vi "Unibot - State Machine Controller.vi"(5 "Up Optimal Gain":dbl[](array[numeric])=[-16.4615, -16.2422, -3.1287, -2.0658], 7 "Setpoint Theta":dbl(knob) scale=-0.1..0.1, 8 "Enable":bool, 9 "Kill":bool, 10 "Setpoint V":dbl(knob) scale=-0.1..0.1, 11 "States":dbl[](array[numeric])=[-0.0012566370614359172, -0.8117875416876026, 0.0, 0.0]) -> (0 "Status":string="Kill", 2 "Control Effort":dbl=-0.1425196371146851)   [LabVIEW 2012]
uses:
  Code/LabVIEW/Real-Time/Demos/cRIO Motor Control/Unibot/Unibot - States.ctl
  <vilib>/addons/Control Design/_Implementation/CD State Feedback Controller (Single Output).vi
  <vilib>/addons/Control Design/_Implementation/NI_CD_Implementation.lvlib
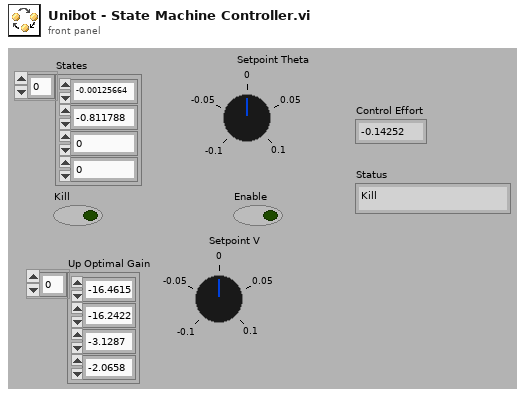
[diagram p1: front panel]
types:
  T1 = typedef "Unibot - States.ctl" = enum16{"Idle", "Balance", "Emergency"}
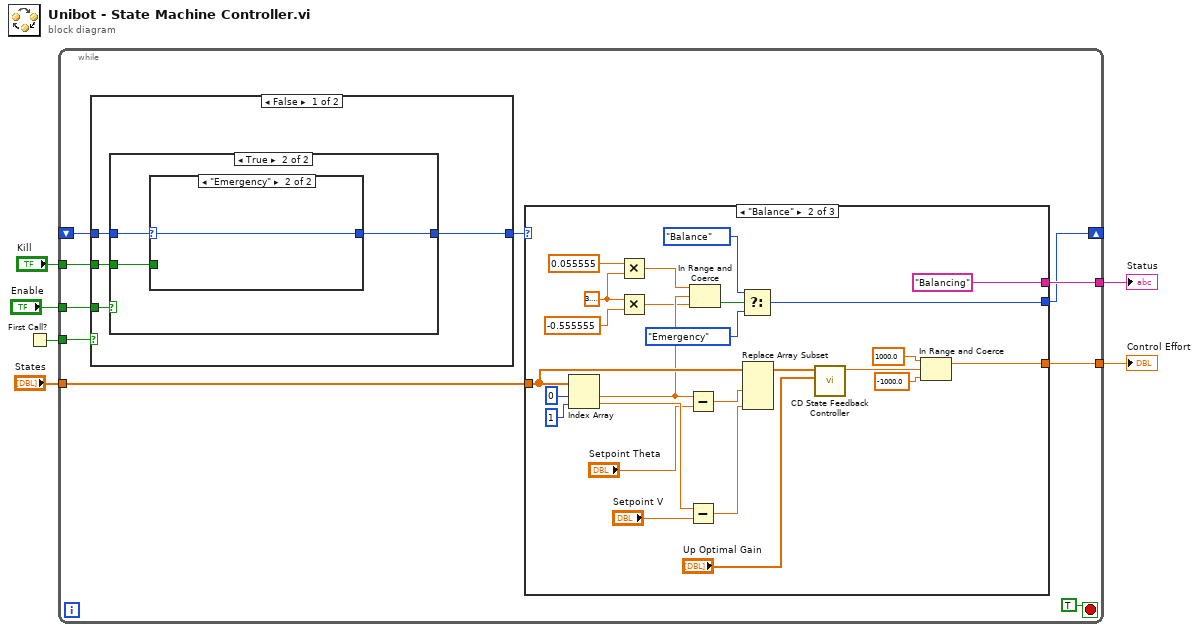
[diagram p0: block diagram]
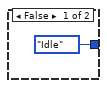
[diagram p2: hidden frame]
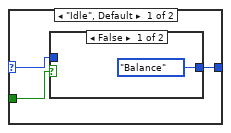
[diagram p3: hidden frame]
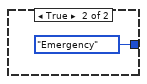
[diagram p4: hidden frame]
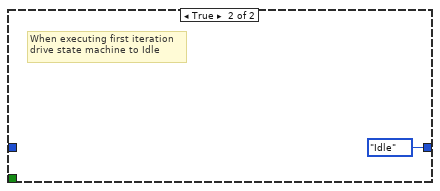
[diagram p5: hidden frame]
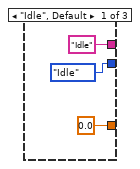
[diagram p6: hidden frame]
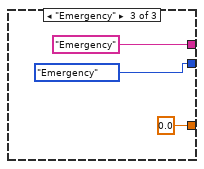
[diagram p7: hidden frame]
diagram:
  n1 = First Call?() -> (First Call?: T/F=w2:bool)
  n2 = while {
    tunnel: "States" -> [w15]
    tunnel: [w11] -> w5
    shift-right: [w10] -> _
    shift-left: _ -> [w12]
    tunnel: [w14] -> w4
    tunnel: "Kill" -> [w13]
    tunnel: w2 -> [w8]
    tunnel: "Enable" -> [w7]
    stop <- TRUE stop-if-true
    n3 = case shown="False" w8 {
      tunnel: w13 -> [w20 _]
      tunnel: w12 -> [w19 _]
      tunnel: [w18 Unibot_-_States."Idle" ("Enum")] -> w9
      tunnel: w7 -> [w17 _]
      frame False {
        n4 = case shown="True" w17 {
          tunnel: w20 -> [_ w24]
          tunnel: [Unibot_-_States."Idle" ("Enum") w23] -> w18
          tunnel: w19 -> [_ w22]
          frame False {
          }
          frame True {
            n5 = case shown="\"Emergency\"" w22 {
              selector: w22 -> [w26 w30]
              tunnel: w24 -> [w27 _]
              tunnel: [w25 w30] -> w23
              frame "Idle", Default {
                n6 = case shown="False" w27 {
                  tunnel: [Unibot_-_States."Balance" ("Enum") Unibot_-_States."Emergency" ("Enum")] -> w25
                  tunnel: w26 -> [_ _]
                  frame False {
                  }
                  frame True {
                  }
                }
              }
              frame "Emergency" {
              }
            }
          }
        }
      }
      frame True {
        # "When executing first iteration\ndrive state machine to Idle"
      }
    }
    n7 = case shown="\"Balance\"" w9 {
      tunnel: w15 -> [_ w52 _]
      tunnel: [0.0 w46 0.0] -> w11
      tunnel: [Unibot_-_States."Idle" ("Enum") w59 Unibot_-_States."Emergency" ("Enum")] -> w10
      tunnel: ["Idle" "Balancing" "Emergency"] -> w14
      frame "Idle", Default {
      }
      frame "Balance" {
        w44 = 3.141592653589793 ("Setpoint")
        n8 = Index Array(array=w52, index #1=0 ("index"), index #2=1 ("index")) -> (element #1=w51:dbl, element #2=w54:dbl)
        n9 = Multiply(x=0.055555, y=w44) -> (x*y=w42:dbl)
        n10 = Multiply(x=w44, y=-0.555555) -> (x*y=w40:dbl)
        n11 = Subtract(x=w51, y="Setpoint Theta") -> (x-y=w55:dbl)
        n12 = Subtract(x=w54, y="Setpoint V") -> (x-y=w53:dbl)
        n13 = In Range and Coerce(upper limit=w42, x=w51, lower limit=w40) -> (In Range?=w39:bool)  [unwired: 1 out]
        n14 = Select(t=Unibot_-_States."Balance" ("Enum"), s=w39, f=Unibot_-_States."Emergency" ("Enum")) -> (s? t:f=w59:T1)
        n15 = Replace Array Subset(array=w52, new element #1=w55, new element #2=w53) -> (w58:dbl[])  [unwired: 2 in]
        n16 = call-poly <vilib>:"CD State Feedback Controller.vi"("Controller Gain"="Up Optimal Gain", "States"=w58) -> ("Controller Action"=w47:dbl)  [unwired: 1 in, 8 out]
        n17 = In Range and Coerce(upper limit=1000.0, x=w47, lower limit=-1000.0) -> (coerced(x)=w46:dbl)  [unwired: 1 out]
      }
      frame "Emergency" {
      }
    }
  }
  "Control Effort" <- w5
  "Status" <- w4
